vi "VI Server_Get RadioButtonsControl Cluster.vi"(7 "Label":string, 8 "error in":errorcluster, 11 "VI Server Cluster":T1) -> (0 "error out":errorcluster, 3 "VI Server Cluster.OUT":T1, 4 "RadioButtonLabels":string[](array[string]))   [LabVIEW 2020, in "VI Server Toolkit LV2013.lvlib"]
doc: "Merges radio Button Controls (Cluster) into VI Server Cluster and returns Radio Button Labels array."
uses:
  VI Server Toolkit LV2013.lvlib
  VI Server_TypeDefs/VI Server_RefsCluster.ctl
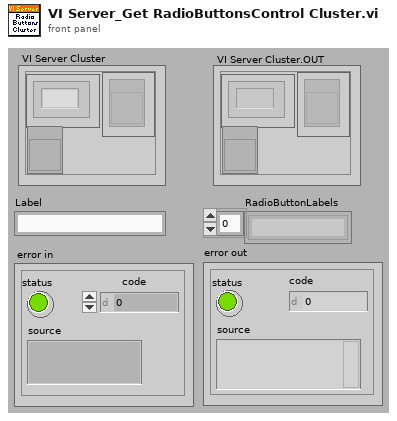
[diagram p1: front panel]
types:
  T1 = typedef "VI Server_RefsCluster.ctl" = cluster{"Labels":string[], "Refs":refnum<vi>[], "VI Ref":refnum<vi>}
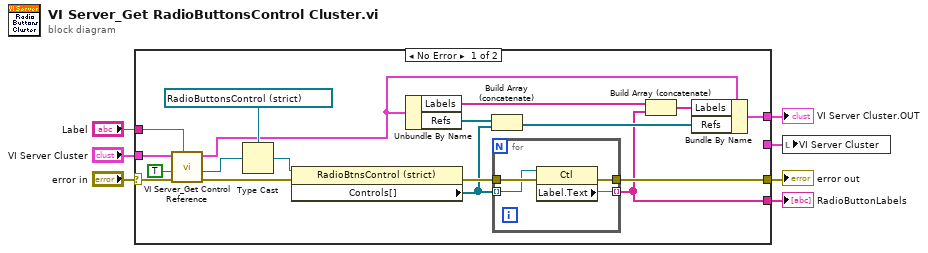
[diagram p0: block diagram]
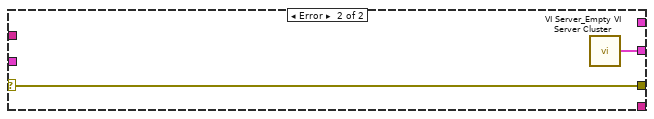
[diagram p2: hidden frame]
diagram:
  n1 = case shown="No Error" "error in" {
    selector: "error in" -> [w10 w31]
    tunnel: "VI Server Cluster" -> [w25 _]
    tunnel: "Label" -> [w24 _]
    tunnel: [w15 w31] -> w5
    tunnel: [w11 _] -> w4
    tunnel: [w9 _] -> w2
    tunnel: [_ w30] -> w1
    frame No Error {
      n2 = call "VI Server_Get Control Reference.vi"("Label"=w24, "error in"=w10, "Single Instance (T)"=TRUE, "VI Server Cluster"=w25) -> ("error out"=w21:errorcluster, "Control Reference (Generic)"=w23:refnum<vi>, "VI Server Cluster.DUP"=w14:T1)  [unwired: 5 out]
      n3 = Type Cast(type=refnum<vi> refnum ("EL.Seat2.MotorSelect"), x=w23) -> (*(type *) &x=w20:refnum<vi>)
      n4 = property class="RadioBtnsControl (strict)"(reference=w20, error in=w21) -> (error out=w19:errorcluster, "Controls[]"=w17:refnum<vi>[])  [unwired: 1 out]
      n5 = Unbundle By Name(w14) -> ("Labels"=w16:string[], "Refs"=w18:refnum<vi>[])
      n6 = Build Array (concatenate)(w18, w17) -> (w12:refnum<vi>[])
      n7 = for {
        tunnel: w17 -> [w28] mode=indexing
        tunnel: w19 -> [w29]
        tunnel: [w27] -> w15
        tunnel: [w26] -> w9 mode=indexing
        n8 = property class="Ctl"(reference=w28, error in=w29) -> (error out=w27:errorcluster, "Label.Text"=w26:string)  [unwired: 1 out]
      }
      n9 = Build Array (concatenate)(w16, w9) -> (w13:string[])
      n10 = Bundle By Name(cluster=w14, "Labels"=w13, "Refs"=w12) -> (w11:T1)
    }
    frame Error {
      n11 = call "VI Server_Empty VI Server Cluster.vi"() -> ("VI Server Cluster"=w30:T1)  [unwired: 7 in]
    }
  }
  "error out" <- w5
  "VI Server Cluster.OUT" <- w4
  "RadioButtonLabels" <- w2
  n12 = local write "VI Server Cluster"(w1) -> ()
